vi "getSpectrometer.vi"(8 "error in (no error)":errorcluster, 10 "Boolean":bool, 11 "SEDSpectrometer in":refnum<class "FiberSpectrograph.lvclass">) -> (0 "error out":errorcluster, 1 "AviableSpec":u8[](array[numeric]), 3 "SEDSpectrometer out":refnum<class "FiberSpectrograph.lvclass">)   [LabVIEW 2016, in "FiberSpectrograph.lvclass"]
uses:
  FiberSpectrograph.lvclass
panel:
  out "DeviceStatus":string[][](table)
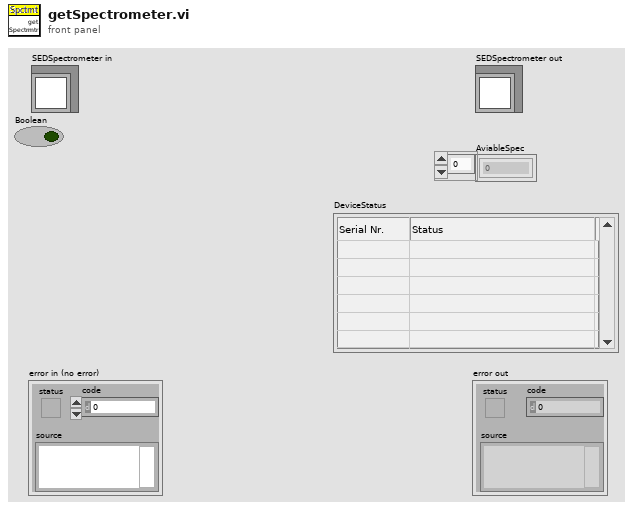
[diagram p1: front panel]
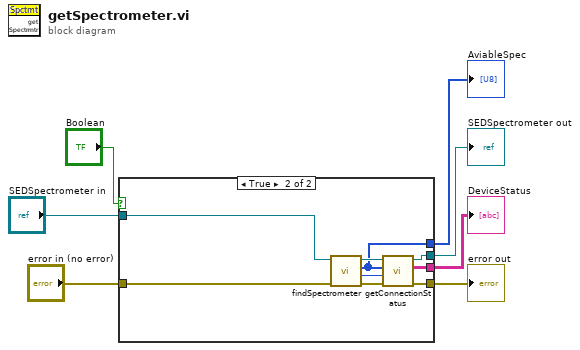
[diagram p0: block diagram]
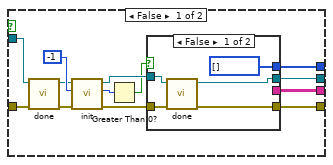
[diagram p2: hidden frame]
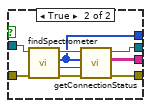
[diagram p3: hidden frame]
diagram:
  n1 = case shown="True" "Boolean" {
    tunnel: [w11 w38] -> w7
    tunnel: [w10 w37] -> w5
    tunnel: [w9 w36] -> w6
    tunnel: "SEDSpectrometer in" -> [w16 w43]
    tunnel: "error in (no error)" -> [w15 w42]
    tunnel: [w8 w35] -> w1
    frame False {
      n2 = call "done.vi"("error in (no error)"=w15, "SEDSpectrometer in"=w16) -> ("error out"=w20:errorcluster, "SEDSpectrometer out"=w18:refnum<class "FiberSpectrograph.lvclass">)  [unwired: 7 in, 1 out]
      n3 = call "init.vi"("error in (no error)"=w20, "Port"=-1, "SEDSpectrometer in"=w18) -> ("error out"=w12:errorcluster, "Output Value"=w17:i32, "SEDSpectrometer out"=w14:refnum<class "FiberSpectrograph.lvclass">)  [unwired: 6 in]
      n4 = Greater Than 0?(x=w17) -> (x > 0?=w13:bool)
      n5 = case shown="False" w13 {
        tunnel: w14 -> [w25 w31]
        tunnel: w12 -> [w24 w30]
        tunnel: [w23 w29] -> w11
        tunnel: [w22 w28] -> w9
        tunnel: [_ w27] -> w10
        tunnel: [u8[] [] ("AviableSpec 2") w26] -> w8
        frame False {
          n6 = call "done.vi"("error in (no error)"=w24, "SEDSpectrometer in"=w25) -> ("error out"=w23:errorcluster, "SEDSpectrometer out"=w22:refnum<class "FiberSpectrograph.lvclass">)  [unwired: 7 in, 1 out]
        }
        frame True {
          n7 = call "findSpectrometer.vi"("error in (no error)"=w30, "SEDSpectrometer in"=w31) -> ("error out"=w34:errorcluster, "NumOfDevices"=w33:i32, "AviableSpec"=w26:u8[], "SEDSpectrometer out"=w32:refnum<class "FiberSpectrograph.lvclass">)  [unwired: 6 in]
          n8 = call "getConnectionStatus.vi"("SEDSpectrometer in"=w32, "AvailableSpectrometer"=w26, "NumOfDevices"=w33, "error in (no error)"=w34) -> ("SEDSpectrometer out"=w28:refnum<class "FiberSpectrograph.lvclass">, "DeviceStatus"=w27:string[][], "error out"=w29:errorcluster)  [unwired: 4 in]
        }
      }
    }
    frame True {
      n9 = call "findSpectrometer.vi"("error in (no error)"=w42, "SEDSpectrometer in"=w43) -> ("error out"=w39:errorcluster, "NumOfDevices"=w40:i32, "AviableSpec"=w35:u8[], "SEDSpectrometer out"=w41:refnum<class "FiberSpectrograph.lvclass">)  [unwired: 6 in]
      n10 = call "getConnectionStatus.vi"("SEDSpectrometer in"=w41, "AvailableSpectrometer"=w35, "NumOfDevices"=w40, "error in (no error)"=w39) -> ("SEDSpectrometer out"=w36:refnum<class "FiberSpectrograph.lvclass">, "DeviceStatus"=w37:string[][], "error out"=w38:errorcluster)  [unwired: 4 in]
    }
  }
  "error out" <- w7
  "SEDSpectrometer out" <- w6
  "DeviceStatus" <- w5
  "AviableSpec" <- w1
